vi "read_write.vi"() -> ()   [LabVIEW 2016]
uses:
  dxl_x86_c.lvlib/dxl_x86_c.lvlib
panel:
  in  "device_name":string="COM1"
  in  "ADDR_PRO_\nPRESENT_POSITION":u16=611
  in  "ADDR_PRO_\nGOAL_POSITION":u16=596
  in  "ADDR_PRO_\nTORQUE_ENABLE":u16=562
  out "protocol_version":dbl=2.0
  out "value : PRO (knob)\npresent position":i32(knob) scale=150000.0..-150000.0
  in  "terminate":bool
  out "port_num":i32
  in  "value : PRO (dial)\ngoal position":i32(knob) scale=150000.0..-150000.0
  in  "dynamixel_id":u8=1
  in  "baud_rate":i32=1000000
  # "/*******************************************************************************\n* Copyright (c) 2016, ROBOTIS CO., LTD.\n* All rights reserved.\n*\n* Redistribution and use in source and binary forms, with or without\n* modification, are permitted provided that the following conditions are met:\n*\n* * Redistributions of source code must retain the above copyright notice, this\n*   list of conditions and the following disclaimer.\n*\n* * Redistributions in binary form must reproduce the above copyright notice,\n*   this list of conditions and the following disclaimer in the documentation\n*   and/or other materials provided with the distribution.\n*\n* * Neither the name of ROBOTIS nor the names of its\n*   contributors may be used to endorse or promote products derived from\n*   this software without specific prior written permission.\n*\n* THIS SOFTWARE IS PROVIDED BY THE COPYRIGHT HOLDERS AND CONTRIBUTORS \"AS IS\"\n* AND ANY EXPRESS OR IMPLIED WARRANTIES, INCLUDING, BUT NOT LIMITED TO, THE\n* IMPLIED WARRANTIES OF MERCHANTABILITY AND FITNESS FOR A PARTICULAR PURPOSE ARE\n* DISCLAIMED. IN NO EVENT SHALL THE COPYRIGHT HOLDER OR CONTRIBUTORS BE LIABLE\n* FOR ANY DIRECT, INDIRECT, INCIDENTAL, SPECIAL, EXEMPLARY, OR CONSEQUENTIAL\n* DAMAGES (INCLUDING, BUT NOT LIMITED TO, PROCUREMENT OF SUBSTITUTE GOODS OR\n* SERVICES; LOSS OF USE, DATA, OR PROFITS; OR BUSINESS INTERRUPTION) HOWEVER\n* CAUSED AND ON ANY THEORY OF LIABILITY, WHETHER IN CONTRACT, STRICT LIABILITY,\n* OR TORT (INCLUDING NEGLIGENCE OR OTHERWISE) ARISING IN ANY WAY OUT OF THE USE\n* OF THIS SOFTWARE, EVEN IF ADVISED OF THE POSSIBILITY OF SUCH DAMAGE.\n*******************************************************************************/\n\n/* Author: Ryu Woon Jung (Leon) */"
  # "Available Dynamixel model on this example : All models using Protocol 2.0\nThis example is designed for using a Dynamixel PRO 54-200, and an USB2DYNAMIXEL.\nTo use another Dynamixel model, such as X series, see their details in E-Manual(support.robotis.com) \n   and edit \"numeric control\"s seen left with \"Edit Text\" tool.\nBe sure that Dynamixel PRO properties are already set as %% ID : 1 / Baudnum : 1 (Baudrate : 57600)\n\n1. Run example by click above \"Run\" button (below \"Edit\" menu).\n2. Drag \"dial\" then you may see the Dynamixel and \"knob\" rotating\n3. To finish the example, press \"terminate\" button."
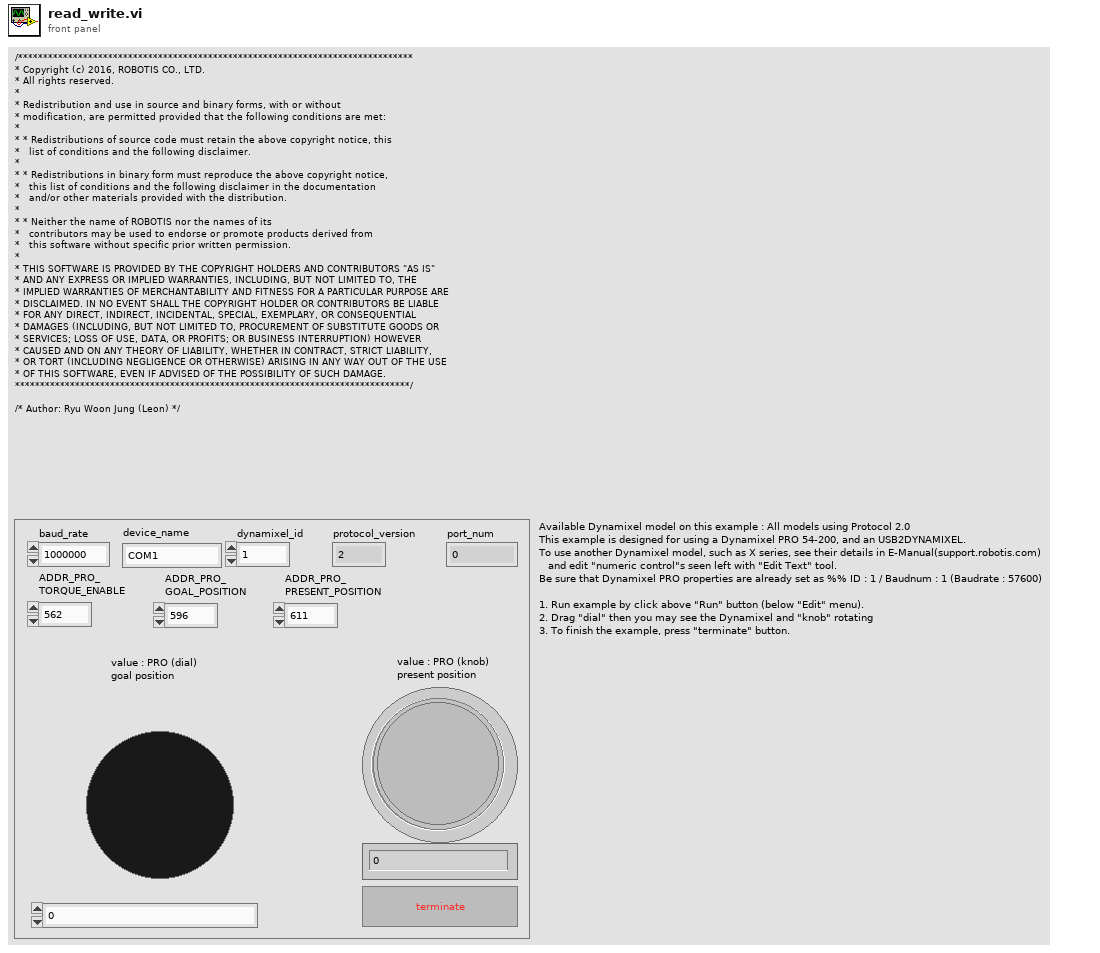
[diagram p1: front panel]
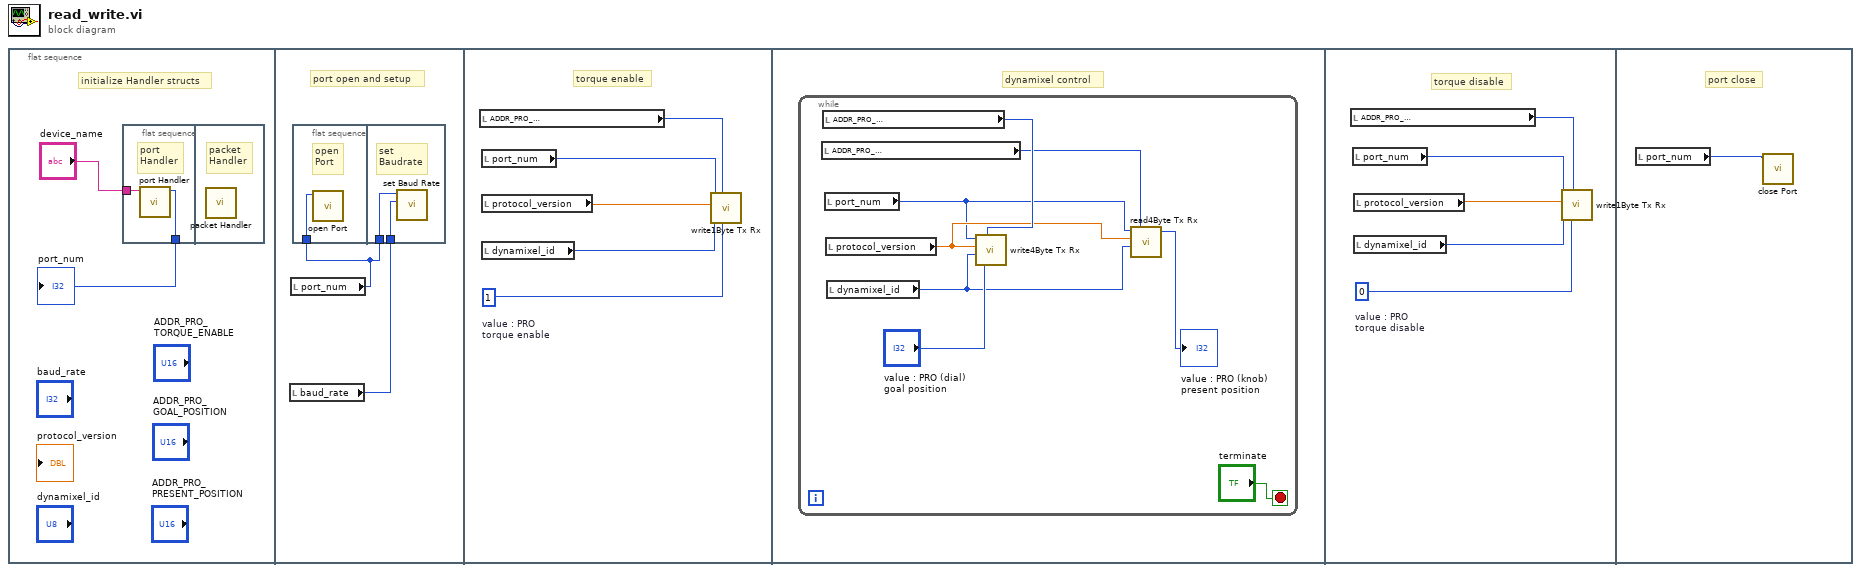
[diagram p0: block diagram]
diagram:
  n1 = flat-sequence {
    frame #0 {
      # "initialize Handler structs"
      n2 = flat-sequence {
        tunnel: [w4] -> w2
        tunnel: "device_name" -> [w3]
        frame #0 {
          # "port\nHandler"
          n3 = call "port Handler.vi"("port_name"=w3) -> ("function return"=w4:i32)  [unwired: 10 in]
        }
        frame #1 {
          # "packet\nHandler"
          n4 = call "packet Handler.vi"() -> ()  [unwired: 12 in]
        }
      }
      "port_num" <- w2
    }
    frame #1 {
      # "port open and setup"
      n5 = local read "baud_rate"() -> (w5:i32)
      n6 = local read "port_num"() -> (w6:i32)
      n7 = flat-sequence {
        tunnel: w6 -> [w7]
        tunnel: w6 -> [w9]
        tunnel: w5 -> [w8]
        frame #0 {
          # "open\nPort"
          n8 = call "open Port.vi"("port_num"=w7) -> ()  [unwired: 10 in, 1 out]
        }
        frame #1 {
          # "set\nBaudrate"
          n9 = call "set Baud Rate.vi"("baudrate"=w8, "port_num"=w9) -> ()  [unwired: 9 in, 1 out]
        }
      }
    }
    frame #2 {
      w14 = 1  # value : PRO torque enable
      # "torque enable"
      n10 = local read "ADDR_PRO_\nTORQUE_ENABLE"() -> (w10:u16)
      n11 = local read "port_num"() -> (w12:i32)
      n12 = local read "protocol_version"() -> (w11:dbl)
      n13 = local read "dynamixel_id"() -> (w13:u8)
      n14 = call "write1Byte Tx Rx.vi"("data"=w14, "address"=w10, "id"=w13, "protocol_version"=w11, "port_num"=w12) -> ()  [unwired: 7 in]
    }
    frame #3 {
      # "dynamixel control"
      n15 = while {
        stop <- "terminate" stop-if-true
        n16 = local read "ADDR_PRO_\nPRESENT_POSITION"() -> (w16:u16)
        n17 = local read "ADDR_PRO_\nGOAL_POSITION"() -> (w21:u16)
        n18 = local read "port_num"() -> (w17:i32)
        n19 = local read "protocol_version"() -> (w18:dbl)
        n20 = local read "dynamixel_id"() -> (w19:u8)
        n21 = call "write4Byte Tx Rx.vi"("data"="value : PRO (dial)\ngoal position", "address"=w21, "id"=w19, "protocol_version"=w18, "port_num"=w17) -> ()  [unwired: 7 in]
        n22 = call "read4Byte Tx Rx.vi"("address"=w16, "id"=w19, "protocol_version"=w18, "port_num"=w17) -> ("function return"=→"value : PRO (knob)\npresent position":u32)  [unwired: 7 in]
      }
    }
    frame #4 {
      w25 = 0  # value : PRO torque disable
      # "torque disable"
      n23 = local read "ADDR_PRO_\nTORQUE_ENABLE"() -> (w23:u16)
      n24 = local read "port_num"() -> (w27:i32)
      n25 = local read "protocol_version"() -> (w24:dbl)
      n26 = local read "dynamixel_id"() -> (w26:u8)
      n27 = call "write1Byte Tx Rx.vi"("data"=w25, "address"=w23, "id"=w26, "protocol_version"=w24, "port_num"=w27) -> ()  [unwired: 7 in]
    }
    frame #5 {
      # "port close"
      n28 = local read "port_num"() -> (w28:i32)
      n29 = call "close Port.vi"("port_num"=w28) -> ()  [unwired: 11 in]
    }
  }
